vi "init.vi"(8 "error in (no error)":errorcluster, 10 "Resource":string, 11 "PsTti in":refnum<class "PsuTti.lvclass">) -> (0 "error out":errorcluster, 3 "PsTti out":refnum<class "PsuTti.lvclass">)   [LabVIEW 2023, in "PsuTti.lvclass"]
doc: "Initialize the instrument by a given resource string or alias name"
uses:
  PsuTti.lvclass
  PsuTti.lvclass/PsuTti.ctl
  PowerSupply.lvclass
  driver/Tti-Pl303Qmd.lvlib
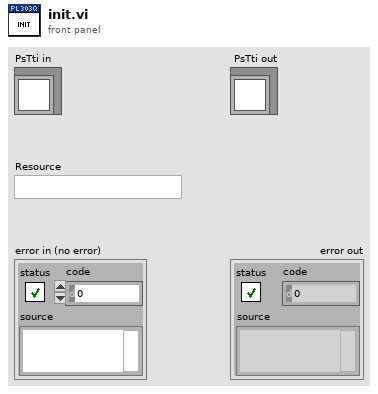
[diagram p1: front panel]
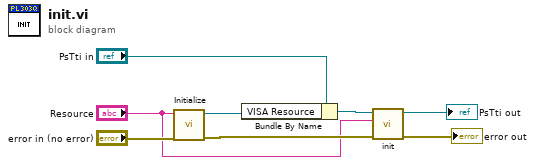
[diagram p0: block diagram]
diagram:
  n1 = call "Initialize.vi"("error in (no error)"="error in (no error)", "VISA resource name"="Resource") -> ("error out"=w3:errorcluster, "VISA resource name out"=w7:refnum<visa-resource-name>)  [unwired: 7 in, 1 out]
  n2 = Bundle By Name(cluster="PsTti in", "VISA Resource"=w7) -> (w6:refnum<class "PsuTti.lvclass">)
  n3 = call-parent "init.vi"("error in (no error)"=w3, "Resource"="Resource", "Instrument in"=w6) -> ("error out"=→"error out":errorcluster, "Instrument out"=→"PsTti out":refnum<class "PsuTti.lvclass">)  [unwired: 7 in]
